vi "SoloWeight.vi"() -> ()   [LabVIEW 2019]
panel:
  out "Weight":string
  in  "delay before read (ms)":u32=500
  in  "Weight VISA resource name":refnum<visa-resource-name>="COM1"
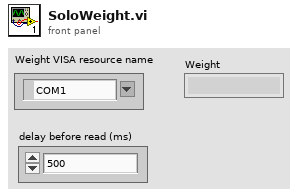
[diagram p1: front panel]
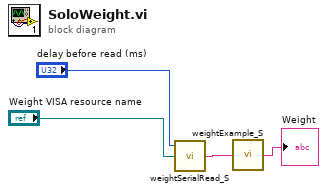
[diagram p0: block diagram]
diagram:
  n1 = call "weightSerialRead_S.vi"("Weight VISA resource name"="Weight VISA resource name", "delay before read (ms)"="delay before read (ms)") -> ("String"=w4:string)  [unwired: 1 in]
  n2 = call "weightExample_S.vi"("weight"=w4) -> ("String"=→"Weight":string)
